vi "NI 9411_task.vi"(6 "divisor":u32=4, 8 "error in":errorcluster, 9 "CI.Freq.Term":tag="/CDRMod7/PFI3", 10 "Counter":string, 11 "MODULE NAME":string="cDAQ_NICOTRAMod5/ctr0") -> (0 "error out":errorcluster, 3 "task out":refnum<k21>)   [LabVIEW 2019]
uses:
  <vilib>/DAQmx/create/channels.llb/DAQmx Create Channel (CI-Frequency).vi
  <resource>/objmgr/daqmx.rc
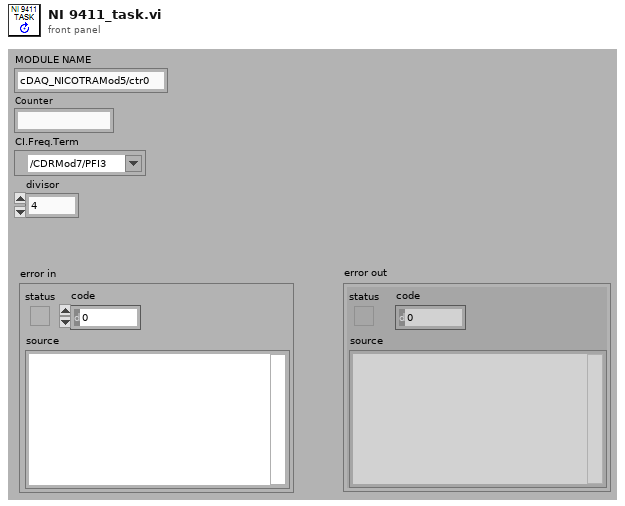
[diagram p1: front panel]
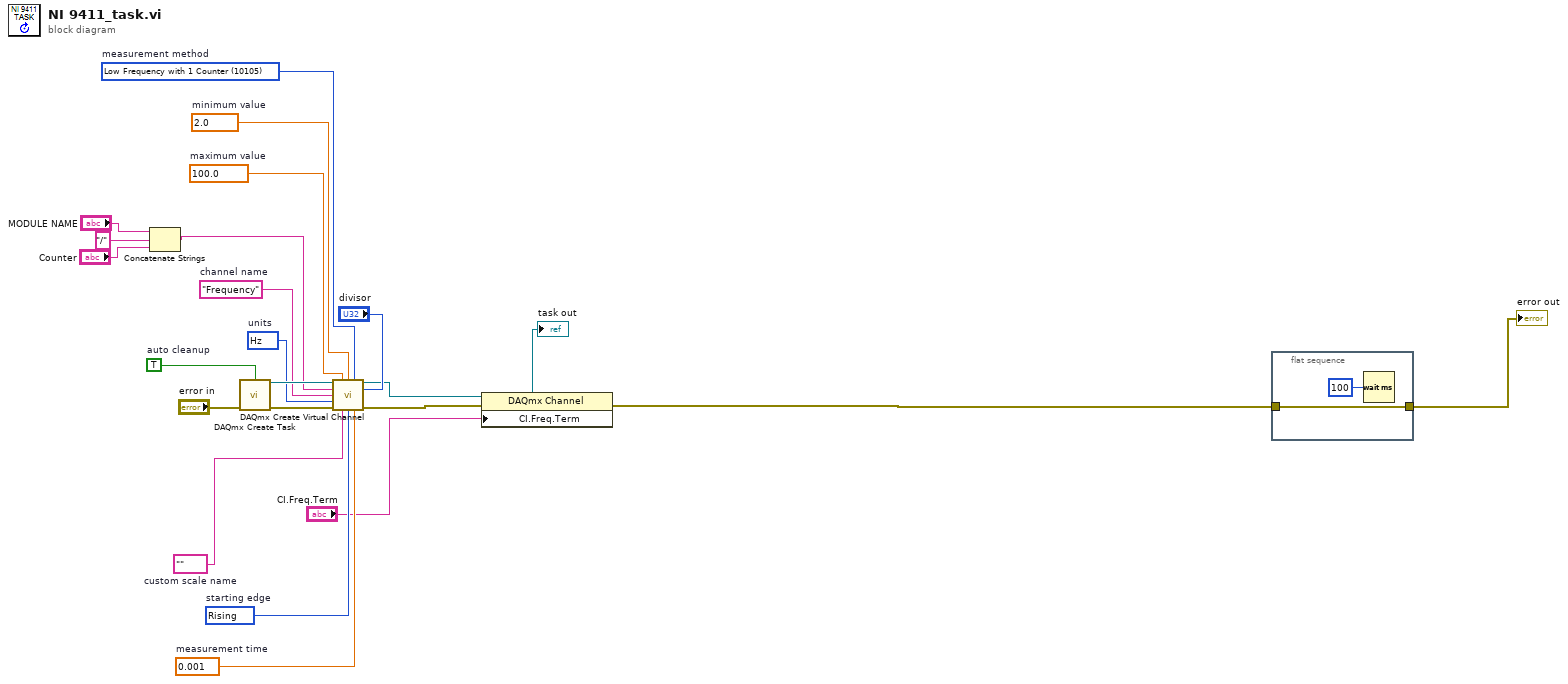
[diagram p0: block diagram]
diagram:
  w9 = tag ""  # custom scale name
  w10 = 10280 items=["Rising"=10280, "Falling"=10171]  # starting edge
  w13 = 10373 items=["Hz"=10373, "Ticks"=10304, "From Custom Scale"=10065]  # units
  w14 = 0.001  # measurement time
  w16 = 10105 items=["Low Frequency with 1 Counter"=10105, "High Frequency with 2 Counters"=10157, "Large Range with 2 Counters"=10205]  # measurement method
  w17 = "Frequency"  # channel name
  w18 = 2.0  # minimum value
  w19 = 100.0  # maximum value
  w21 = TRUE  # auto cleanup
  n1 = Concatenate Strings("MODULE NAME", "/" ("string"), "Counter") -> (w3:string)
  n2 = call <vilib>:"DAQmx Create Task.vi"("auto cleanup"=w21, "error in"="error in") -> ("task out"=w20:refnum<k21>, "error out"=w22:errorcluster)  [unwired: 12 in]
  n3 = call-poly <vilib>:"DAQmx Create Virtual Channel.vi"("task in"=w20, "maximum value"=w19, "minimum value"=w18, "measurement method"=w16, "counter"=w3, "divisor"="divisor", "name to assign"=w17, "units"=w13, "error in"=w22, "custom scale name"=w9, "starting edge"=w10, "measurement time"=w14) -> ("task out"=w12:refnum<k21>, "error out"=w8:errorcluster)  [unwired: 2 in]
  n4 = property class="DAQmx Channel"(reference=w12, error in=w8, "CI.Freq.Term"="CI.Freq.Term") -> (reference out=→"task out":refnum<k21>, error out=w6:errorcluster)
  n5 = flat-sequence {
    tunnel: w6 -> [w25]
    tunnel: [w25] -> w5
    frame #0 {
      n6 = Wait (ms)(milliseconds to wait=u32 100) -> ()  [unwired: 1 out]
    }
  }
  "error out" <- w5
